vi "mxwScript_Cmnd2Str_changeObjectToLocal.vi"(8 "error in (no error)":errorcluster, 11 "data":variant) -> (0 "error out":errorcluster, 3 "outputString":string)   [LabVIEW 2017]
uses:
  codeGenAPISupport.llb/cgAPI_mxwScript_ConvertToLocalInfo.ctl
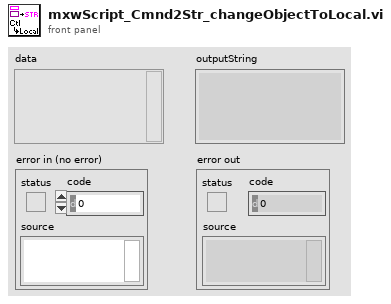
[diagram p1: front panel]
types:
  T1 = typedef "cgAPI_mxwScript_ConvertToLocalInfo.ctl" = cluster{"name":string, "index":i32, "targetName":string, "targetIndex":i32, "toLocalType":enum16{"Auto", "Read", "Write"}}
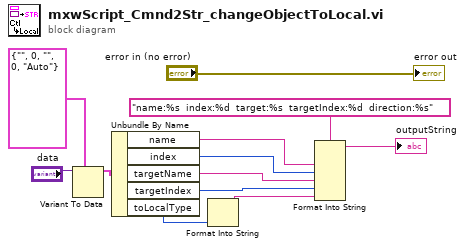
[diagram p0: block diagram]
diagram:
  n1 = Variant To Data(type=T1 {"name"="", "index"=0, "targetName"="", "targetIndex"=0, "toLocalType"=enum."Auto"} ("convertToLocalInfo"), Variant="data") -> (data=w9:T1)  [unwired: 1 in, 1 out]
  n2 = Unbundle By Name(w9) -> ("name"=w6:string, "index"=w5:i32, "targetName"=w4:string, "targetIndex"=w3:i32, "toLocalType"=w8:enum16{"Auto", "Read", "Write"})
  n3 = Format Into String(w8) -> (resulting string=w2:string)  [unwired: 3 in, 1 out]
  n4 = Format Into String(format string="name:%s  index:%d  target:%s  targetIndex:%d  direction:%s", w6, w5, w4, w3, w2) -> (resulting string=→"outputString":string)  [unwired: 2 in, 1 out]
  "error out" <- "error in (no error)"
